vi "Error 5003.vi"(8 "error in (no error)":errorcluster) -> (0 "error out":errorcluster)   [LabVIEW 2019, in "gRPC Scripting Tools.lvlib"]
uses:
  gRPC Scripting Tools.lvlib
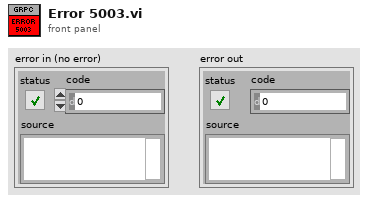
[diagram p1: front panel]
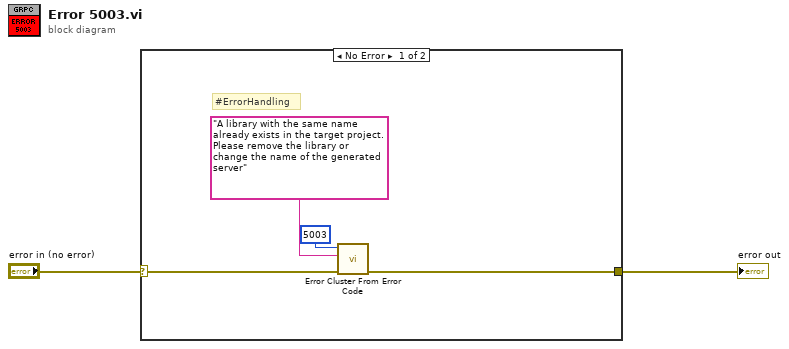
[diagram p0: block diagram]
diagram:
  n1 = case shown="No Error" "error in (no error)" {
    selector: "error in (no error)" -> [w3 w7]
    tunnel: [w6 w7] -> w2
    frame No Error {
      # "#ErrorHandling"
      n2 = call <vilib>:"Error Cluster From Error Code.vi"("error in (no error)"=w3, "error message (\"\")"="A library with the same name already exists in the target project. Please remove the library or change the name of the generated server" ("error message (\"\")"), "error code (0)"=5003) -> ("error out"=w6:errorcluster)  [unwired: 6 in]
    }
    frame Error {
    }
  }
  "error out" <- w2
